vi "Moving_Statistic_Set_Window.vi"(8 "error in (no error)":errorcluster, 10 "Window":i32, 11 "Moving_Statistic in":refnum<class "Moving_Statistic.lvclass">) -> (0 "error out":errorcluster, 3 "Moving_Statistic out":refnum<class "Moving_Statistic.lvclass">)   [LabVIEW 2021, in "Moving_Statistic.lvclass"]
uses:
  Moving_Statistic.lvclass
  Moving_Statistic.lvclass/Moving_Statistic.ctl
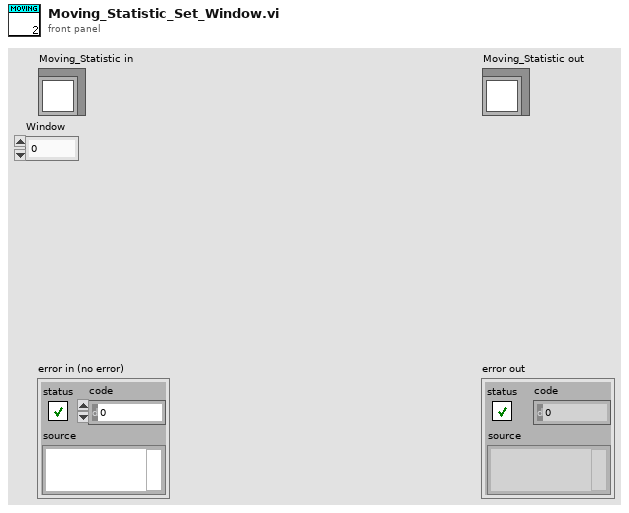
[diagram p1: front panel]
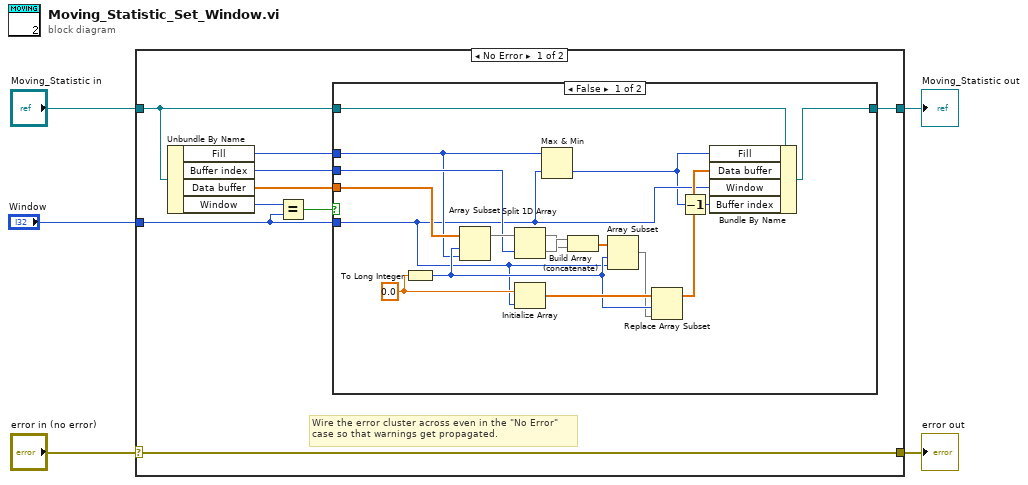
[diagram p0: block diagram]
diagram:
  n1 = case shown="No Error" "error in (no error)" {
    selector: "error in (no error)" -> [w14 w34]
    tunnel: [w14 w34] -> w4
    tunnel: [w13 w33] -> w2
    tunnel: "Moving_Statistic in" -> [w12 w33]
    tunnel: "Window" -> [w7 _]
    frame No Error {
      # "Wire the error cluster across even in the \"No Error\"\ncase so that warnings get propagated."
      n2 = Unbundle By Name(w12) -> ("Fill"=w9:i32, "Buffer index"=w10:i32, "Data buffer"=w11:dbl[], "Window"=w8:i32)
      n3 = Equal?(x=w8, y=w7) -> (x = y?=w6:bool)
      n4 = case shown="False" w6 {
        tunnel: [w28 w32] -> w13
        tunnel: w12 -> [w27 w32]
        tunnel: w11 -> [w31 _]
        tunnel: w10 -> [w22 _]
        tunnel: w9 -> [w18 _]
        tunnel: w7 -> [w17 _]
        frame False {
          w24 = 0.0 ("element")
          n5 = To Long Integer(number=w24) -> (32bit integer=w20:i32)
          n6 = Array Subset(array=w31, index=w20, length=w18) -> (w23:dbl[])
          n7 = Split 1D Array(array=w23, index=w22) -> (first subarray=w29:dbl[], second subarray=w30:dbl[])
          n8 = Initialize Array(w24, w17) -> (w26:dbl[])
          n9 = Max & Min(x=w18, y=w17) -> (min(x,y)=w16:i32)  [unwired: 1 out]
          n10 = Build Array (concatenate)(w30, w29) -> (w21:dbl[])
          n11 = Array Subset(array=w21, index=w20, length=w17) -> (w19:dbl[])
          n12 = Replace Array Subset(array=w26, new element=w19, index=w20) -> (w25:dbl[])
          n13 = Decrement(x=w16) -> (x-1=w15:i32)
          n14 = Bundle By Name(cluster=w27, "Fill"=w16, "Data buffer"=w25, "Window"=w17, "Buffer index"=w15) -> (w28:refnum<class "Moving_Statistic.lvclass">)
        }
        frame True {
        }
      }
    }
    frame Error {
    }
  }
  "error out" <- w4
  "Moving_Statistic out" <- w2
